vi "LoadFromFileDisplay.vi"() -> ()   [LabVIEW 2009]
doc: "Use this template to simulate the acquisition of data by reading data from a file.\nNote: LabVIEW enables automatic error handling by default for VIs you create from this template."
panel:
  out "Current 3":dynamicdata(graph)
  out "Current 2":dynamicdata(graph)
  out "Current":dynamicdata(graph)
  in  "stop":bool
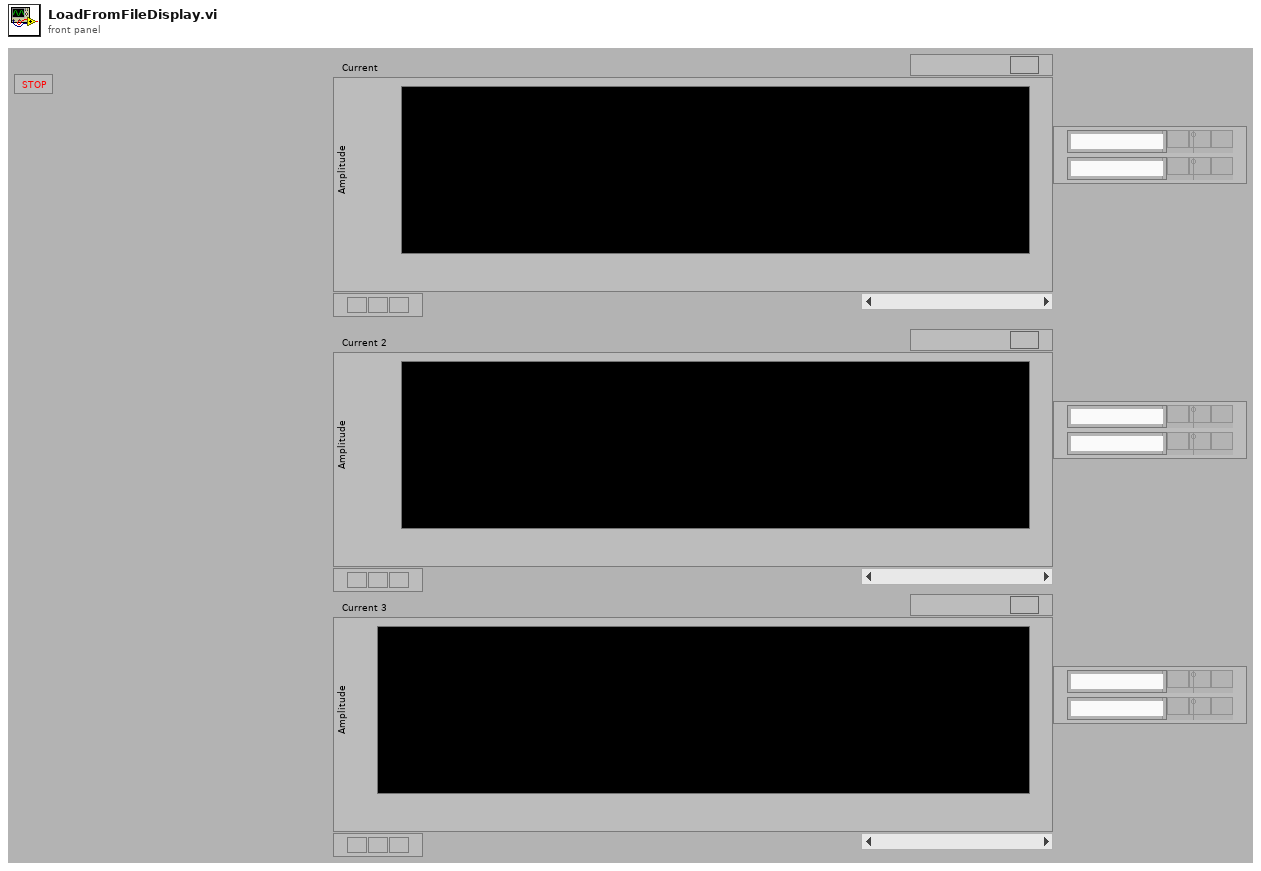
[diagram p1: front panel]
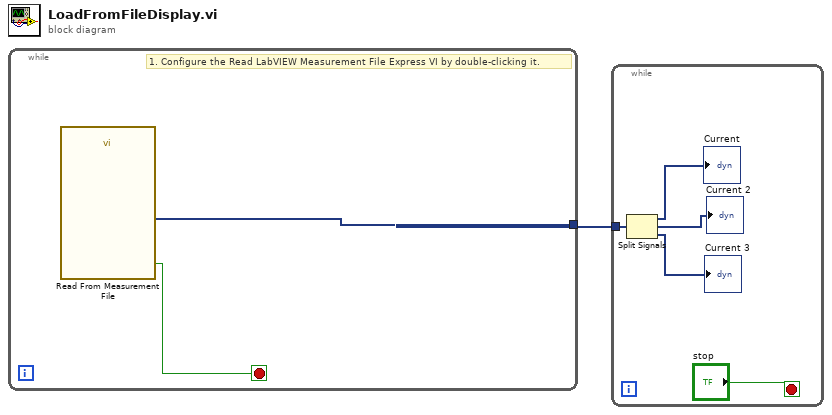
[diagram p0: block diagram]
diagram:
  n1 = while {
    tunnel: [w3] -> w1
    stop <- w2 stop-if-true
    # "1. Configure the Read LabVIEW Measurement File Express VI by double-clicking it."
    n2 = call "Read From Measurement File"() -> ("Signals"=w3:dynamicdata, "EOF?"=w2:bool)  [unwired: 6 in, 4 out]
  }
  n3 = while {
    tunnel: w1 -> [w8]
    stop <- "stop" stop-if-true
    n4 = Split Signals(w8) -> (→"Current":dynamicdata, →"Current 2":dynamicdata, →"Current 3":dynamicdata)  [unwired: 3 in]
  }
